vi "choose com ports.vi"(9 "Default COM ports IN":string[](array[string]), 10 "Default IMAGING shutter":string="PXI1Slot3/port0/line0", 11 "optional modules":string[](array[string])) -> (1 "Default COM ports OUT":string[](array[string]))   [LabVIEW 2012]
doc: "SciScan 1.2 160622"
uses:
  GFG/GFGstringGet.vi
  GFG/GFG library.lvlib
  <resource>/objmgr/daqmx.rc
panel:
  in  "shutter.DO":u16(ring) caption="IMAGING shutter port" items=["Dev1/port0/line0", "Dev1/port0/line1", "Dev1/port0/line2", "Dev1/port0/line3", "Dev1/port0/line4", "Dev1/port0/line5", "Dev1/port0/line6", "Dev1/port0/line7", "Dev2/port0/line0", "Dev2/port0/line1", "Dev2/port0/line2", "Dev2/port0/line3", "Dev2/port0/line4", "Dev2/port0/line5", "Dev2/port0/line6", "Dev2/port0/line7", "Dev2/port1/line0", "Dev2/port1/line1", "Dev2/port1/line2", "Dev2/port1/line3", "Dev2/port1/line4", "Dev2/port1/line5", "Dev2/port1/line6", "Dev2/port1/line7", "Dev2/port2/line0", "Dev2/port2/line1", "Dev2/port2/line2", "Dev2/port2/line3", "Dev2/port2/line4", "Dev2/port2/line5", "Dev2/port2/line6", "Dev2/port2/line7", "PXI1Slot3/port0/line0", "PXI1Slot3/port0/line1", "PXI1Slot3/port0/line2", "PXI1Slot3/port0/line3", "PXI1Slot3/port0/line4", "PXI1Slot3/port0/line5", "PXI1Slot3/port0/line6", "PXI1Slot3/port0/line7", "PXI1Slot3/port1/line0", "PXI1Slot3/port1/line1", "PXI1Slot3/port1/line2", "PXI1Slot3/port1/line3", "PXI1Slot3/port1/line4", "PXI1Slot3/port1/line5", "PXI1Slot3/port1/line6", "PXI1Slot3/port1/line7", "PXI1Slot3/port2/line0", "PXI1Slot3/port2/line1", "PXI1Slot3/port2/line2", "PXI1Slot3/port2/line3", "PXI1Slot3/port2/line4", "PXI1Slot3/port2/line5", "PXI1Slot3/port2/line6", "PXI1Slot3/port2/line7", "PXI1Slot4/port0/line0", "PXI1Slot4/port0/line1", "PXI1Slot4/port0/line2", "PXI1Slot4/port0/line3", "PXI1Slot4/port0/line4", "PXI1Slot4/port0/line5", "PXI1Slot4/port0/line6", "PXI1Slot4/port0/line7", "PXI1Slot4/port1/line0", "PXI1Slot4/port1/line1", "PXI1Slot4/port1/line2", "PXI1Slot4/port1/line3", "PXI1Slot4/port1/line4", "PXI1Slot4/port1/line5", "PXI1Slot4/port1/line6", "PXI1Slot4/port1/line7", "PXI1Slot4/port2/line0", "PXI1Slot4/port2/line1", "PXI1Slot4/port2/line2", "PXI1Slot4/port2/line3", "PXI1Slot4/port2/line4", "PXI1Slot4/port2/line5", "PXI1Slot4/port2/line6", "PXI1Slot4/port2/line7", "PXI1Slot5/port0/line0", "PXI1Slot5/port0/line1", "PXI1Slot5/port0/line2", "PXI1Slot5/port0/line3", "PXI1Slot5/port0/line4", "PXI1Slot5/port0/line5", "PXI1Slot5/port0/line6", "PXI1Slot5/port0/line7", "PXI1Slot5/port1/line0", "PXI1Slot5/port1/line1", "PXI1Slot5/port1/line2", "PXI1Slot5/port1/line3", "PXI1Slot5/port1/line4", "PXI1Slot5/port1/line5", "PXI1Slot5/port1/line6", "PXI1Slot5/port1/line7", "PXI1Slot5/port2/line0", "PXI1Slot5/port2/line1", "PXI1Slot5/port2/line2", "PXI1Slot5/port2/line3", "PXI1Slot5/port2/line4", "PXI1Slot5/port2/line5", "PXI1Slot5/port2/line6", "PXI1Slot5/port2/line7"]
  in  "stop":bool
  in  "MM.port":u16(ring)
  in  "PMT34.port":u16(ring)
  in  "PMT12.port":u16(ring)
  in  "MIC.port":u16(ring)
  in  "stage.port":u16(ring)
  # "Configure COM ports\nand Imaging Shutter"
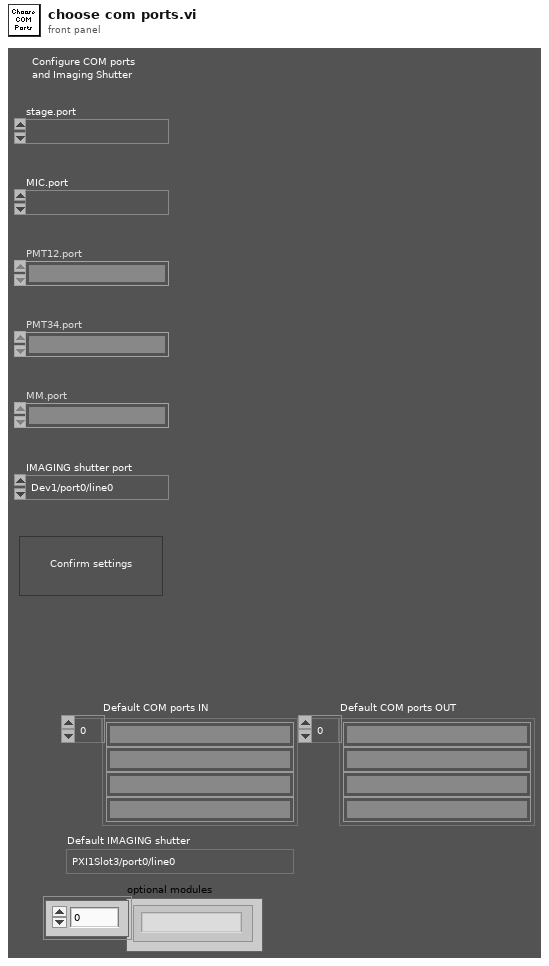
[diagram p1: front panel]
types:
  T1 = enum8{"Enabled", "Disabled", "Disabled and Grayed Out"}
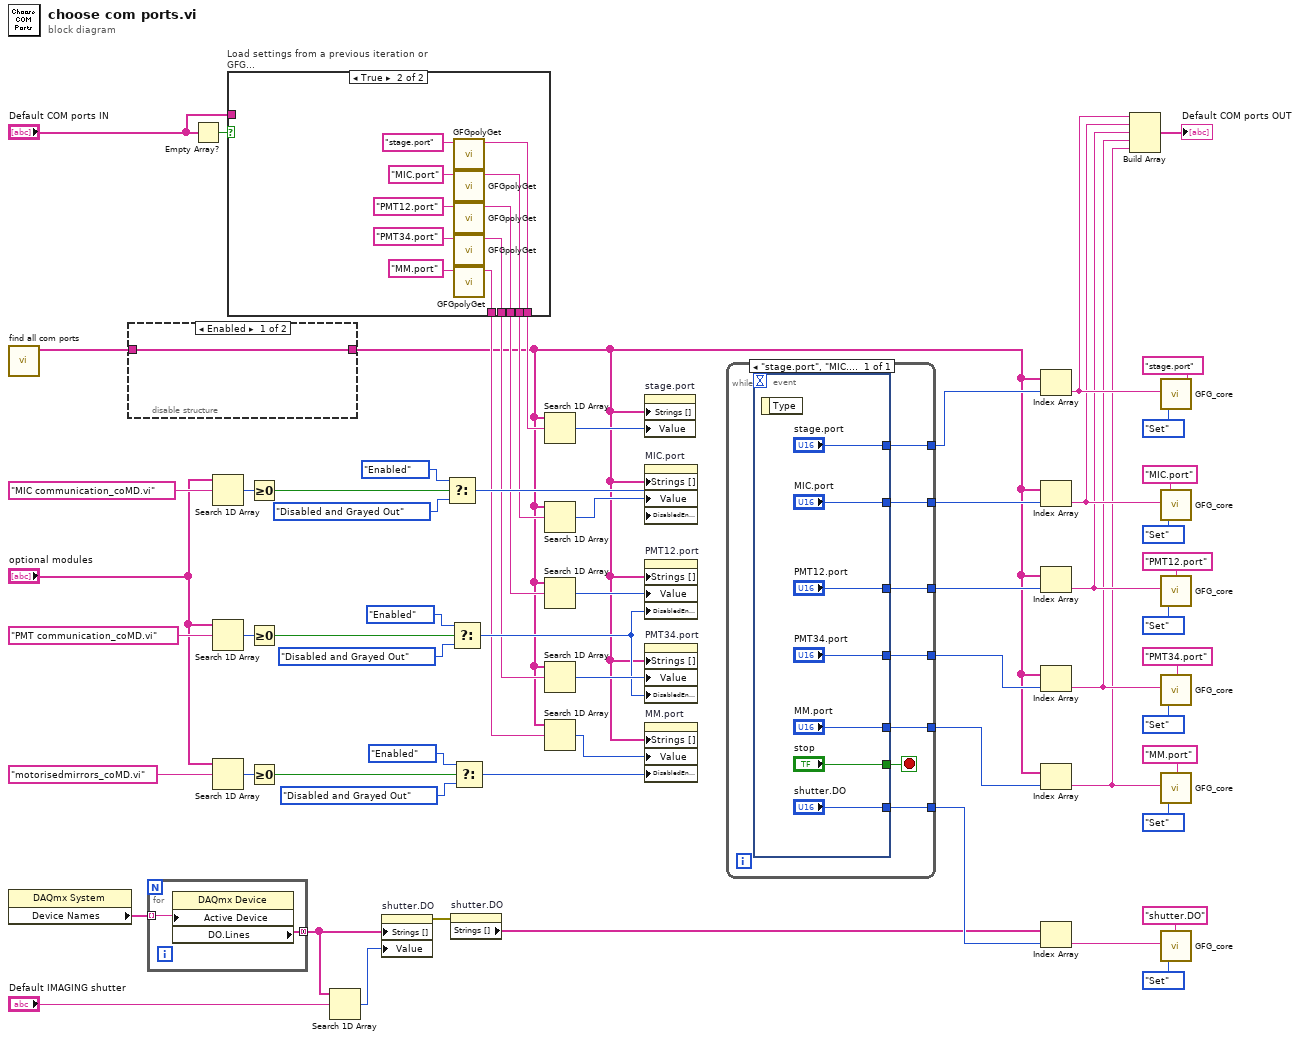
[diagram p0: block diagram]
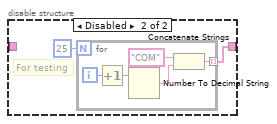
[diagram p2: hidden frame]
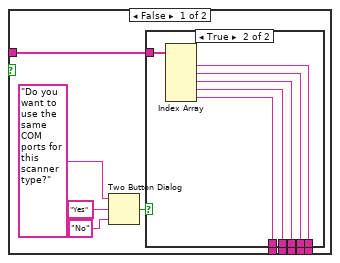
[diagram p3: hidden frame]
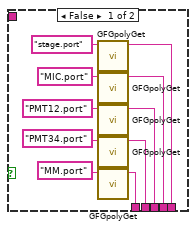
[diagram p4: hidden frame]
diagram:
  n1 = call "find all com ports.vi"() -> ("com ports array"=w2:string[])  [unwired: 11 in]
  n2 = property class="DAQmx System"() -> ("Device Names"=w46:tag[])  [unwired: 2 in, 2 out]
  n3 = disable-structure shown="Enabled" {
    disable-tunnel: w2 -> [w65 _]
    disable-tunnel: [w65 w66] -> w1
    frame Enabled {
    }
    frame Disabled {
      # "For testing"
      n4 = for {
        N: 25 -> [_]
        tunnel: [w70] -> w66 mode=indexing
        i -> [w69]
        n5 = Increment(x=w69) -> (x+1=w68:i32)
        n6 = Number To Decimal String(number=w68) -> (decimal integer string=w71:string)  [unwired: 1 in]
        n7 = Concatenate Strings("COM" ("string"), w71) -> (w70:string)
      }
    }
  }
  n8 = for {
    tunnel: w46 -> [w73] mode=indexing
    tunnel: [w74] -> w16 mode=concatenating
    n9 = property class="DAQmx Device"("Active Device"=w73) -> ("DO.Lines"=w74:tag[])  [unwired: 2 in, 2 out]
  }
  n10 = Empty Array?(array="Default COM ports IN") -> (empty?=w15:bool)
  n11 = Search 1D Array(1D array="optional modules", element="MIC communication_coMD.vi") -> (index of element=w40:i32)  [unwired: 1 in]
  n12 = Search 1D Array(1D array="optional modules", element="PMT communication_coMD.vi") -> (index of element=w34:i32)  [unwired: 1 in]
  n13 = Search 1D Array(1D array="optional modules", element="motorisedmirrors_coMD.vi") -> (index of element=w30:i32)  [unwired: 1 in]
  n14 = case "Load settings from a previous iteration or GFG..." shown="True" w15 {
    tunnel: "Default COM ports IN" -> [w80 _]
    tunnel: [w79 w102] -> w7
    tunnel: [w78 w103] -> w6
    tunnel: [w77 w104] -> w5
    tunnel: [w76 w105] -> w4
    tunnel: [w75 w106] -> w3
    frame False {
      n15 = Two Button Dialog(message="Do you want to use the same COM ports for this scanner type?", 1:"No" ("F button name (\"Cancel\")"), 2:"Yes" ("T button name (\"OK\")")) -> (T button?=w81:bool)
      n16 = case shown="True" w81 {
        tunnel: w80 -> [_ w100]
        tunnel: [w93 w99] -> w79
        tunnel: [w91 w98] -> w78
        tunnel: [w87 w97] -> w77
        tunnel: [w86 w96] -> w76
        tunnel: [w85 w95] -> w75
        frame False {
          n17 = call-poly "GFGpolyGet.vi"("Variable Name in"="stage.port") -> ("String"=w93:string)  [unwired: 9 in, 1 out]
          n18 = call-poly "GFGpolyGet.vi"("Variable Name in"="MIC.port") -> ("String"=w91:string)  [unwired: 9 in, 1 out]
          n19 = call-poly "GFGpolyGet.vi"("Variable Name in"="PMT12.port") -> ("String"=w87:string)  [unwired: 9 in, 1 out]
          n20 = call-poly "GFGpolyGet.vi"("Variable Name in"="PMT34.port") -> ("String"=w86:string)  [unwired: 9 in, 1 out]
          n21 = call-poly "GFGpolyGet.vi"("Variable Name in"="MM.port") -> ("String"=w85:string)  [unwired: 9 in, 1 out]
        }
        frame True {
          n22 = Index Array(array=w100) -> (element #1=w99:string, element #2=w98:string, element #3=w97:string, element #4=w96:string, element #5=w95:string)  [unwired: 5 in]
        }
      }
    }
    frame True {
      n23 = call-poly "GFGpolyGet.vi"("Variable Name in"="stage.port") -> ("String"=w102:string)  [unwired: 9 in, 1 out]
      n24 = call-poly "GFGpolyGet.vi"("Variable Name in"="MIC.port") -> ("String"=w103:string)  [unwired: 9 in, 1 out]
      n25 = call-poly "GFGpolyGet.vi"("Variable Name in"="PMT12.port") -> ("String"=w104:string)  [unwired: 9 in, 1 out]
      n26 = call-poly "GFGpolyGet.vi"("Variable Name in"="PMT34.port") -> ("String"=w105:string)  [unwired: 9 in, 1 out]
      n27 = call-poly "GFGpolyGet.vi"("Variable Name in"="MM.port") -> ("String"=w106:string)  [unwired: 9 in, 1 out]
    }
  }
  n28 = Greater Or Equal To 0?(x=w40) -> (x >= 0?=w37:bool)
  n29 = Greater Or Equal To 0?(x=w34) -> (x >= 0?=w32:bool)
  n30 = Greater Or Equal To 0?(x=w30) -> (x >= 0?=w27:bool)
  n31 = Search 1D Array(1D array=w16, element="Default IMAGING shutter") -> (index of element=w20:i32)  [unwired: 1 in]
  n32 = property on="shutter.DO" class="Ring (strict)"("Strings []"=w16, "Value"=w20) -> (error out=w23:errorcluster)  [unwired: 2 in, 1 out]
  n33 = Select(t=T1."Enabled" ("Disabled"), s=w37, f=T1."Disabled and Grayed Out" ("Disabled")) -> (s? t:f=w18:T1)
  n34 = property on="shutter.DO" class="Ring (strict)"(error in=w23) -> ("Strings []"=w22:string[])  [unwired: 1 in, 2 out]
  n35 = Select(t=T1."Enabled" ("Disabled"), s=w32, f=T1."Disabled and Grayed Out" ("Disabled")) -> (s? t:f=w17:T1)
  n36 = Select(t=T1."Enabled" ("Disabled"), s=w27, f=T1."Disabled and Grayed Out" ("Disabled")) -> (s? t:f=w24:T1)
  n37 = Search 1D Array(1D array=w1, element=w7) -> (index of element=w49:i32)  [unwired: 1 in]
  n38 = Search 1D Array(1D array=w1, element=w6) -> (index of element=w19:i32)  [unwired: 1 in]
  n39 = Search 1D Array(1D array=w1, element=w5) -> (index of element=w48:i32)  [unwired: 1 in]
  n40 = Search 1D Array(1D array=w1, element=w4) -> (index of element=w47:i32)  [unwired: 1 in]
  n41 = Search 1D Array(1D array=w1, element=w3) -> (index of element=w25:i32)  [unwired: 1 in]
  n42 = property on="stage.port" class="Ring (strict)"("Strings []"=w1, "Value"=w49) -> ()  [unwired: 2 in, 2 out]
  n43 = property on="MIC.port" class="Ring (strict)"("Strings []"=w1, "Value"=w19, "DisabledEnum"=w18) -> ()  [unwired: 2 in, 2 out]
  n44 = property on="PMT12.port" class="Ring (strict)"("Strings []"=w1, "Value"=w48, "DisabledEnum"=w17) -> ()  [unwired: 2 in, 2 out]
  n45 = property on="PMT34.port" class="Ring (strict)"("Strings []"=w1, "Value"=w47, "DisabledEnum"=w17) -> ()  [unwired: 2 in, 2 out]
  n46 = property on="MM.port" class="Ring (strict)"("Strings []"=w1, "Value"=w25, "DisabledEnum"=w24) -> ()  [unwired: 2 in, 2 out]
  n47 = while {
    tunnel: [w117] -> w56
    tunnel: [w116] -> w53
    tunnel: [w115] -> w52
    tunnel: [w114] -> w51
    tunnel: [w113] -> w50
    tunnel: [w111] -> w45
    stop <- w112 stop-if-true
    n48 = event shown="[0] \"stage.port\", \"MIC.port\", \"PMT12.port\", \"PMT34.port\", \"MM.port\", \"stop\", \"shutter.DO\": Value Change" {
      selector: _ -> [_]
      dyn-events: _ -> [_]
      timeout: _ -> [_]
      tunnel: ["stage.port"] -> w117
      tunnel: ["MIC.port"] -> w116
      tunnel: ["PMT12.port"] -> w115
      tunnel: ["PMT34.port"] -> w114
      tunnel: ["MM.port"] -> w113
      tunnel: ["stop"] -> w112
      tunnel: ["shutter.DO"] -> w111
      event "stage.port", "MIC.port", "PMT12.port", "PMT34.port", "MM.port", "stop", "shutter.DO": Value Change {
        n49 = event-data() -> ()  [unwired: 1 in, 1 out]
      }
    }
  }
  n50 = Index Array(array=w1, index=w56) -> (element=w14:string)
  n51 = Index Array(array=w1, index=w53) -> (element=w13:string)
  n52 = Index Array(array=w1, index=w52) -> (element=w12:string)
  n53 = Index Array(array=w1, index=w51) -> (element=w11:string)
  n54 = Index Array(array=w1, index=w50) -> (element=w10:string)
  n55 = Index Array(array=w22, index=w45) -> (element=w43:string)
  n56 = Build Array(w14, w13, w12, w11, w10) -> (→"Default COM ports OUT":string[])
  n57 = call "GFG_core.vi"("Variable Name in"="stage.port", "Variant in"=w14, "Action"=enum16{"Init", "Set", "Get", "Clear"}."Set") -> ()  [unwired: 10 in, 7 out]
  n58 = call "GFG_core.vi"("Variable Name in"="MIC.port", "Variant in"=w13, "Action"=enum16{"Init", "Set", "Get", "Clear"}."Set") -> ()  [unwired: 10 in, 7 out]
  n59 = call "GFG_core.vi"("Variable Name in"="PMT12.port", "Variant in"=w12, "Action"=enum16{"Init", "Set", "Get", "Clear"}."Set") -> ()  [unwired: 10 in, 7 out]
  n60 = call "GFG_core.vi"("Variable Name in"="PMT34.port", "Variant in"=w11, "Action"=enum16{"Init", "Set", "Get", "Clear"}."Set") -> ()  [unwired: 10 in, 7 out]
  n61 = call "GFG_core.vi"("Variable Name in"="MM.port", "Variant in"=w10, "Action"=enum16{"Init", "Set", "Get", "Clear"}."Set") -> ()  [unwired: 10 in, 7 out]
  n62 = call "GFG_core.vi"("Variable Name in"="shutter.DO", "Variant in"=w43, "Action"=enum16{"Init", "Set", "Get", "Clear"}."Set") -> ()  [unwired: 10 in, 7 out]
